vi "灰度直方图分析.vi"() -> ()   [LabVIEW 2018]
uses:
  <vilib>/vision/NI_Vision_Development_Module.lvlib
panel:
  out "error out":errorcluster
  out "Standard  Deviation":sgl format="%.2f"
  out "Mean Value":sgl format="%.2f"
  out "Histogram Graph":T1 {"Incremental Value" format="%.2f"; "Starting Value" format="%.2f"}
  out "Image":T2(plugin-control)
  in  "路径":path
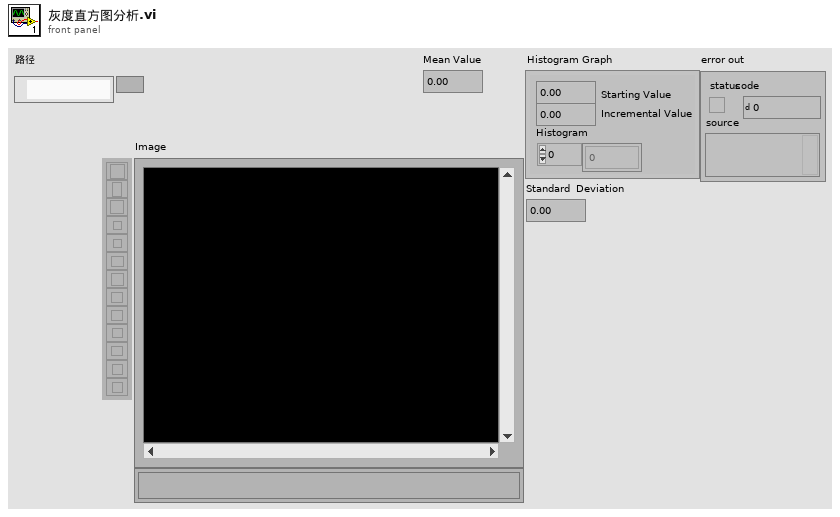
[diagram p1: front panel]
types:
  T1 = cluster{"Starting Value":sgl, "Incremental Value":sgl, "Histogram":u32[]}
  T2 = typedef "IMAQ Image.ctl" = refnum<image>
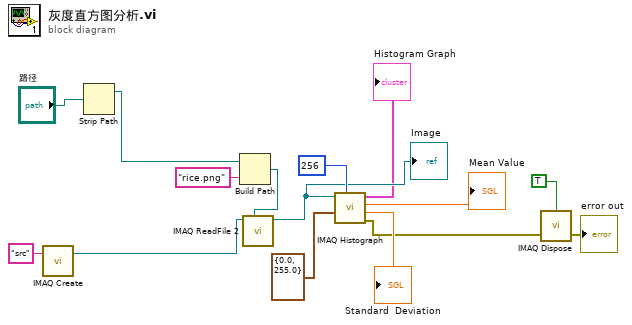
[diagram p0: block diagram]
diagram:
  n1 = call "IMAQ Create"("Image Name"="src") -> ("New Image"=w11:T2)  [unwired: 4 in, 1 out]
  n2 = Strip Path(path="路径") -> (stripped path=w15:path)  [unwired: 1 out]
  n3 = Build Path(base path=w15, name or relative path="rice.png" ("名称或相对路径")) -> (appended path=w13:path)
  n4 = call "IMAQ ReadFile 2"("File Path"=w13, "Image"=w11) -> ("Image Out"=w7:T2)  [unwired: 5 in, 4 out]
  "Image" <- w7
  n5 = call "IMAQ Histograph"("Number of Classes"=256, "Interval Range"=cluster{"Minimum":sgl, "Maximum":sgl} {"Minimum"=0.0, "Maximum"=255.0}, "Image"=w7) -> ("error out"=w3:errorcluster, "Standard  Deviation"=→"Standard  Deviation":sgl, "Mean Value"=→"Mean Value":sgl, "Histogram Graph"=→"Histogram Graph":T1)  [unwired: 5 in]
  n6 = call "IMAQ Dispose"("All Images? (No)"=TRUE, "error in (no error)"=w3) -> ("error out"=→"error out":errorcluster)  [unwired: 4 in]
